vi "Replace or Append Test Data DVR.vi"(8 "error in (no error)":errorcluster, 11 "TopLevel Out in":T1) -> (0 "error out":errorcluster, 2 "CsvPath":path, 3 "TopLevel Out out":T1)   [LabVIEW 2011]
uses:
  Controls/Top Level Control.ctl
  <vilib>/NI/AMC/Message Queue.ctl
  <vilib>/NI/AMC/Message.ctl
  <vilib>/NI/Tools/Keyed Array/KeyedArray.ctl
  Controls/ListBox Test Record.ctl
  Controls/DVR of CSV Tests Data.ctl
  Controls/CSVs Tests Data.ctl
  Controls/Test Column Data.ctl
  Controls/Options DVR.ctl
  Controls/Options.ctl
  <vilib>/NI/Tools/Keyed Array/Tools_KeyedArray.lvlib
  <vilib>/NI/AMC/AMC.lvlib
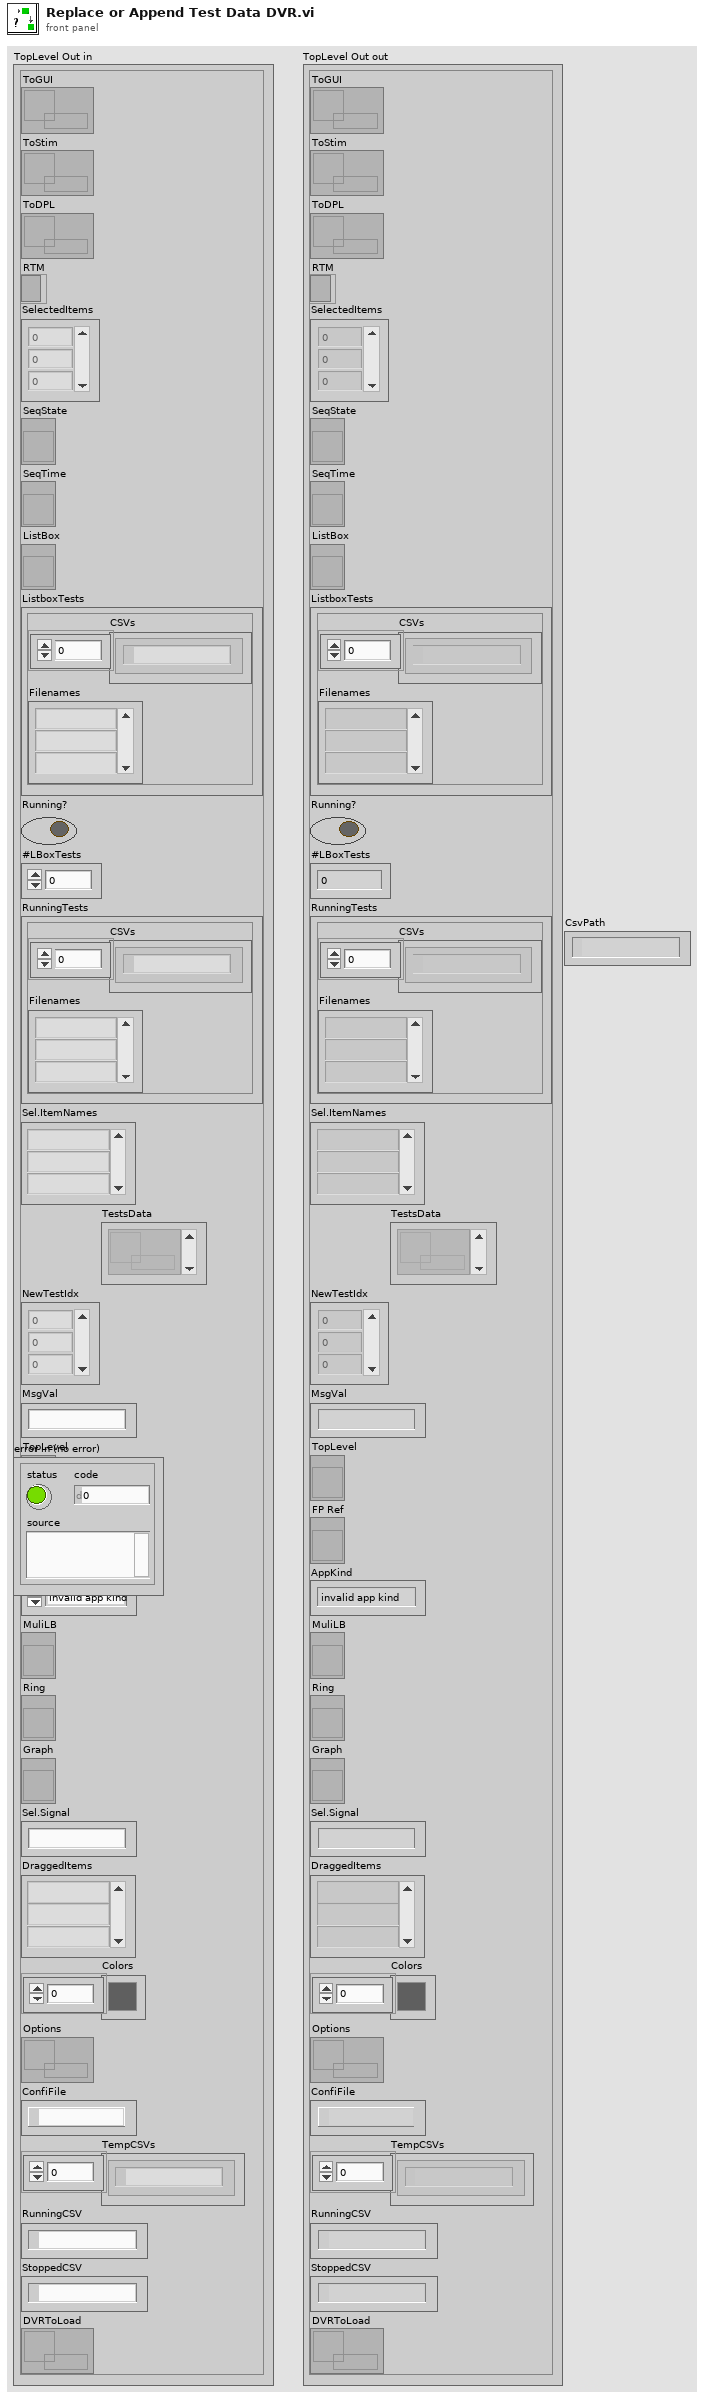
[diagram p1: front panel]
types:
  T1 = typedef "Top Level Control.ctl" = cluster{"ToGUI":T2, "ToStim":T2, "ToDPL":T2, "RTM":refnum<k9>, "SelectedItems":i32[], "SeqState":refnum<vi>, "SeqTime":refnum<vi>, "ListBox":refnum<vi>, "ListboxTests":T3, "Running?":bool, "#LBoxTests":i32, "RunningTests":T3, "Sel.ItemNames":string[], "TestsData":T4[], "NewTestIdx":i32[], "MsgVal":string, "TopLevel":refnum<vi>, "FP Ref":refnum<vi>, "AppKind":enum32{"invalid app kind", "Development System", "Run Time System", "Student Edition", "Embedded LabVIEW", "Evaluation", "Custom"}, "MuliLB":refnum<vi>, "Ring":refnum<vi>, "Graph":refnum<vi>, "Sel.Signal":string, "DraggedItems":string[], "Colors":u32[], "Options":T5, "ConfiFile":path, "TempCSVs":path[], "RunningCSV":path, "StoppedCSV":path, "DVRToLoad":T4}
  T2 = typedef "AMC.lvlib/Message Queue.ctl" = refnum<queue>
  T3 = typedef "ListBox Test Record.ctl" = cluster{"CSVs":path[], "Filenames":string[]}
  T4 = typedef "DVR of CSV Tests Data.ctl" = refnum<data-value>
  T5 = typedef "Options DVR.ctl" = refnum<data-value>
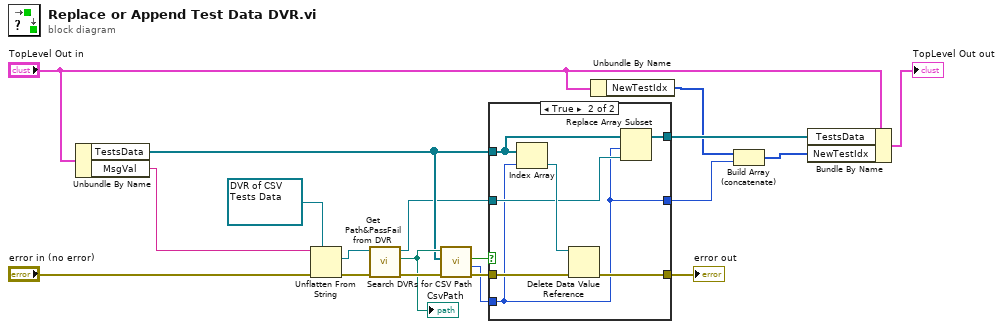
[diagram p0: block diagram]
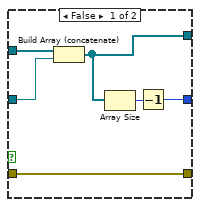
[diagram p2: hidden frame]
diagram:
  n1 = Unbundle By Name("TopLevel Out in") -> ("TestsData"=w11:T4[], "MsgVal"=w5:string)
  n2 = Unflatten From String(type=T4 refnum ("data value reference"), binary string=w5, error in (no error)="error in (no error)") -> (value=w16:T4, error out=w15:errorcluster)  [unwired: 2 in, 1 out]
  n3 = call "Get Path&PassFail from DVR.vi"("error in (no error)"=w15, "Data Value Reference in"=w16) -> ("error out"=w14:errorcluster, "CsvPath"=w13:path, "Data Value Reference out"=w8:T4)  [unwired: 5 in, 2 out]
  "CsvPath" <- w13
  n4 = call "Search DVRs for CSV Path.vi"("error in (no error)"=w14, "DVRs"=w11, "CsvPath"=w13) -> ("error out"=w12:errorcluster, "Idx"=w7:i32, "Found?"=w6:bool)  [unwired: 5 in, 1 out]
  n5 = case shown="True" w6 {
    tunnel: w12 -> [w25 w32]
    tunnel: w11 -> [w24 w30]
    tunnel: [w25 w29] -> w10
    tunnel: [w22 w28] -> w9
    tunnel: w8 -> [w23 w27]
    tunnel: w7 -> [_ w26]
    tunnel: [w20 w26] -> w2
    frame False {
      n6 = Build Array (concatenate)(w24, w23) -> (w22:T4[])
      n7 = Array Size(array=w22) -> (size(s)=w21:i32)
      n8 = Decrement(x=w21) -> (x-1=w20:i32)
    }
    frame True {
      n9 = Index Array(array=w30, index=w26) -> (element=w31:T4)
      n10 = Delete Data Value Reference(data value reference=w31, error in=w32) -> (error out=w29:errorcluster)  [unwired: 1 out]
      n11 = Replace Array Subset(array=w30, new element=w27, index=w26) -> (w28:T4[])
    }
  }
  "error out" <- w10
  n12 = Unbundle By Name("TopLevel Out in") -> ("NewTestIdx"=w3:i32[])
  n13 = Build Array (concatenate)(w3, w2) -> (w1:i32[])
  n14 = Bundle By Name(cluster="TopLevel Out in", "TestsData"=w9, "NewTestIdx"=w1) -> (→"TopLevel Out out":T1)
